vi "Update Data.vi"(3 "Data IN":T1={"PDFTable ref"=refnum, "columnWidth (points)"=[], "Borders"={"Row Borders [ ]"=[], "Last Row"={"Column Borders [ ]"=[], "Line"={"Thickness"=0.5, "Color"=0}}, "Row Back Ground color"={"color"=16777225, "at each"=0.0}}, "Image to Add with path[ ]"=[], "Image to Add with refnum[ ]"=[], "Update"=enum."Others"} caption="Data" {"Image to Add with path[ ]"."Scale" format="%#_g %"}) -> (0 "Data change?":bool, 1 "Data OUT":T1={"PDFTable ref"=refnum, "columnWidth (points)"=[], "Borders"={"Row Borders [ ]"=[], "Last Row"={"Column Borders [ ]"=[], "Line"={"Thickness"=0.5, "Color"=0}}, "Row Back Ground color"={"color"=16777225, "at each"=0.0}}, "Image to Add with path[ ]"=[], "Image to Add with refnum[ ]"=[], "Update"=enum."Others"} caption="Data" {"Image to Add with path[ ]"."Scale" format="%#_g %"})   [LabVIEW 2012]
uses:
  C:/Users/MaxCorp/Documents/GitHub/TopView/DLL/itextsharp.dll
  GitHub/TopView/DLL/itextsharp.dll
  Image Scale.ctl
  Cell Border.ctl
  <userlib>/Exaprom PDF/Controls/PDF Table Xcontrol/Data.ctl
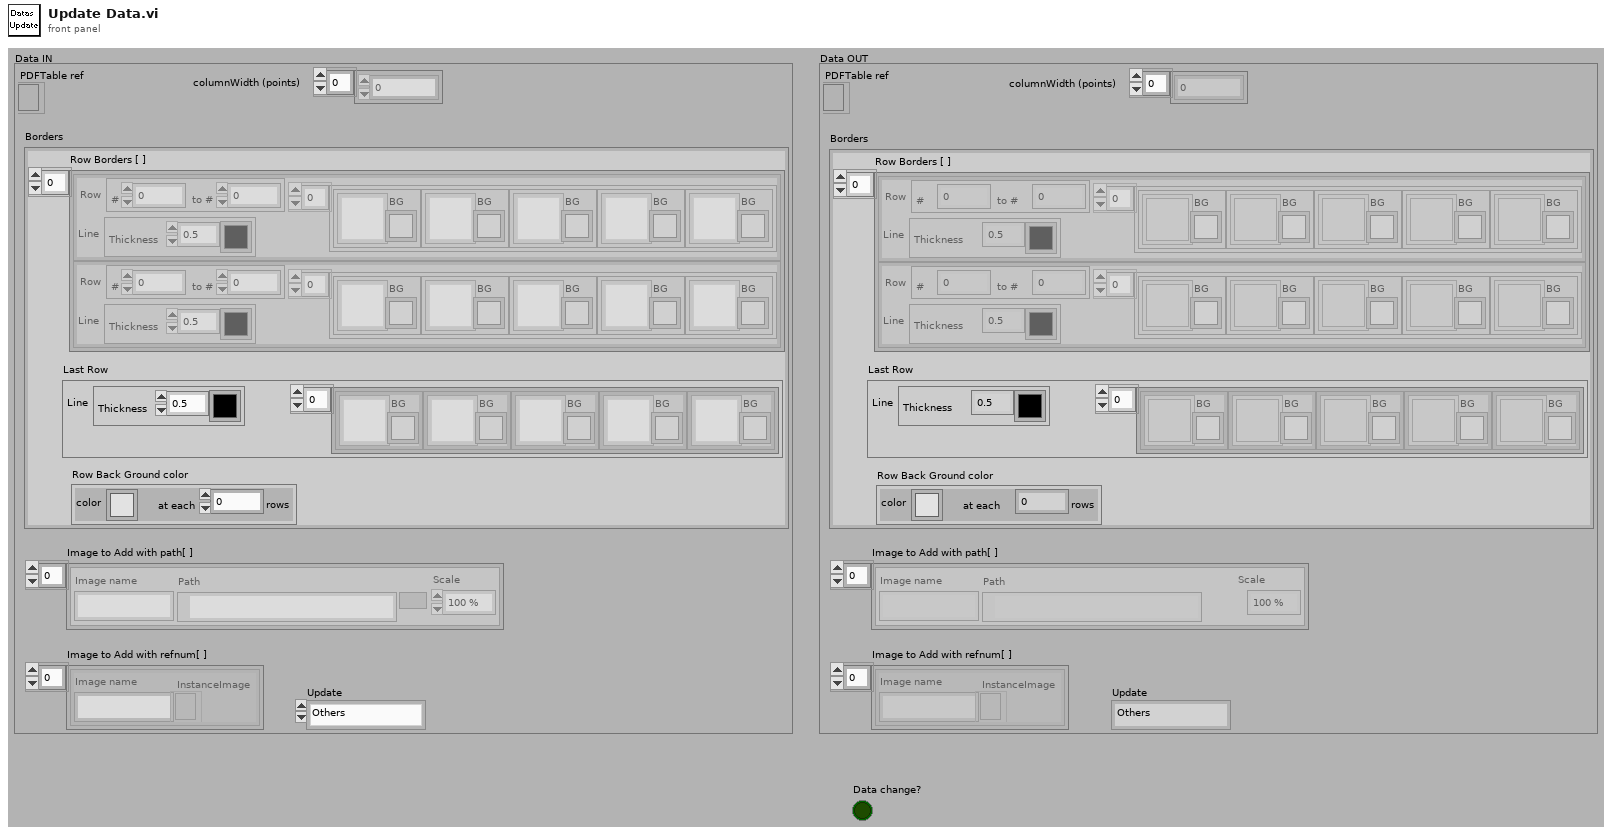
[diagram p1: front panel]
types:
  T1 = typedef "PDF Table XControl.xctl/Data.ctl" = cluster{"PDFTable ref":refnum<k24>, "columnWidth (points)":sgl[], "Borders":cluster{"Row Borders [ ]":cluster{"Column Borders [ ]":cluster{"Cell Border":T2, "BG":u32}[], "Line":cluster{"Thickness":sgl, "Color":u32}, "Row":cluster{"#":u16, "to #":i16}}[], "Last Row":cluster{"Column Borders [ ]":cluster{"Cell Border":T2, "BG":u32}[], "Line":cluster{"Thickness":sgl, "Color":u32}}, "Row Back Ground color":cluster{"color":u32, "at each":dbl}}, "Image to Add with path[ ]":cluster{"Image name":string, "Path":path, "Scale":T3}[], "Image to Add with refnum[ ]":cluster{"Image name":string, "InstanceImage":refnum<k24>}[], "Update":enum16{"Others", "Borders", "Images List"}}
  T2 = typedef "Cell Border.ctl" = u16
  T3 = typedef "Image Scale.ctl" = sgl
  T4 = cluster{"Image name":string, "InstanceImage":refnum<k24>}[]
  T5 = cluster{"Image name":string, "Path":path, "Scale":T3}[]
  T6 = cluster{"Image name":string, "GetInstance":refnum<k24>}
  T7 = cluster{"Image name":string, "GetInstance":refnum<k24>}[]
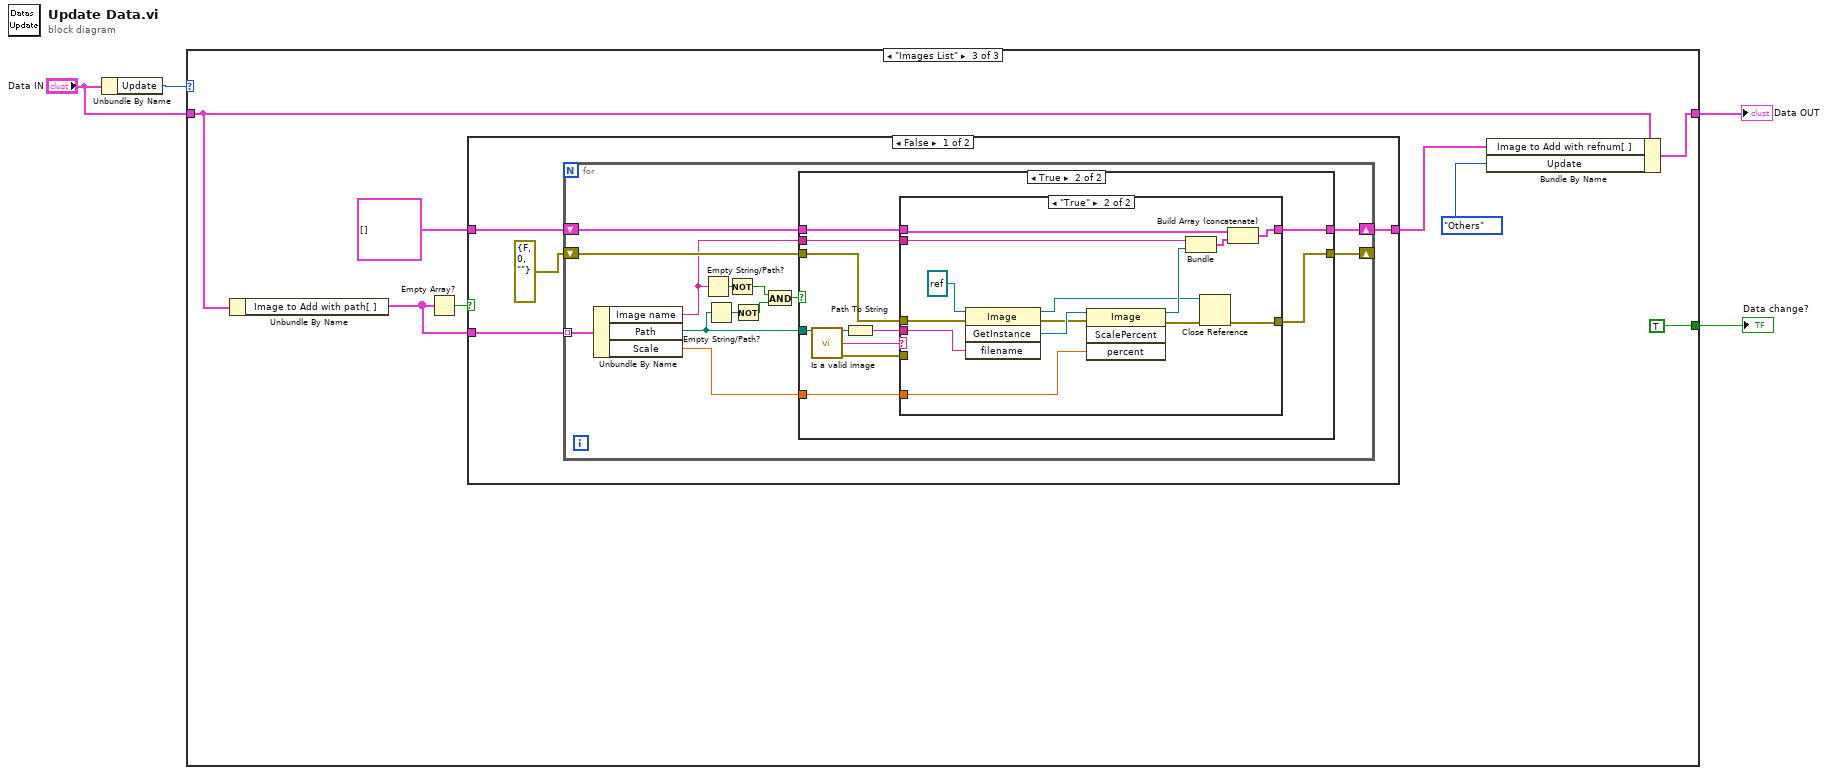
[diagram p0: block diagram]
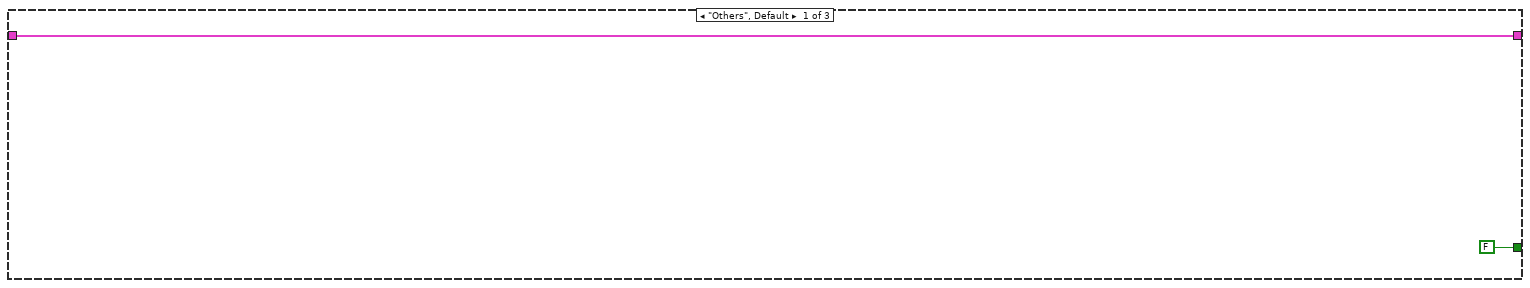
[diagram p2: hidden frame]
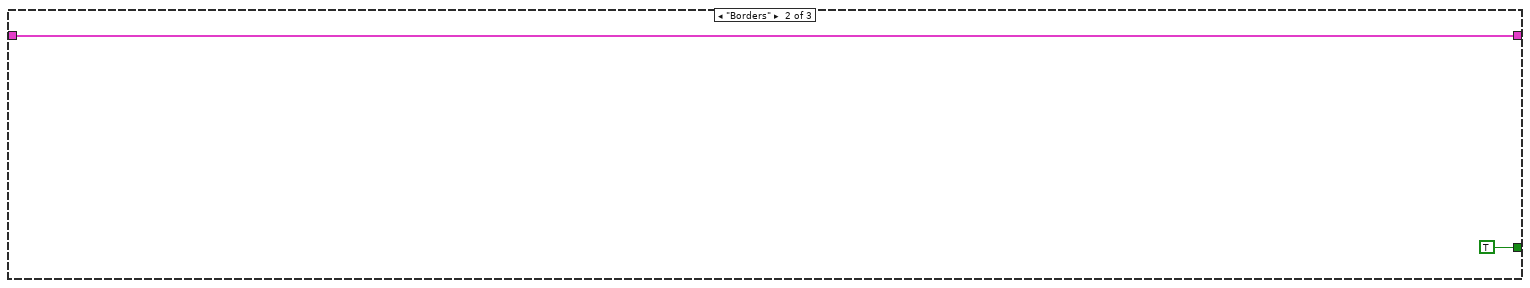
[diagram p3: hidden frame]
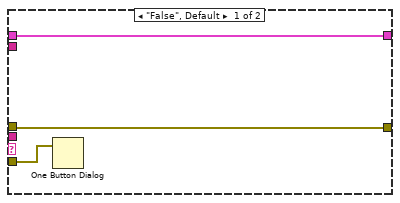
[diagram p5: hidden frame]
diagram:
  n1 = Unbundle By Name("Data IN") -> ("Update"=w4:enum16{"Others", "Borders", "Images List"})
  n2 = case shown="\"Images List\"" w4 {
    tunnel: "Data IN" -> [w6 w8 w12]
    tunnel: [w6 w8 w14] -> w2
    tunnel: [FALSE ("Data change?") TRUE ("Data change?") TRUE ("Data change?")] -> w1
    frame "Others", Default {
    }
    frame "Borders" {
    }
    frame "Images List" {
      n3 = Unbundle By Name(w12) -> ("Image to Add with path[ ]"=w11:T5)
      n4 = Empty Array?(array=w11) -> (empty?=w15:bool)
      n5 = case shown="False" w15 {
        tunnel: w11 -> [w20 _]
        tunnel: T4 [] ("Image to Add [ ]") -> [w19 w64]
        tunnel: [w18 w64] -> w13
        frame False {
          n6 = for {
            tunnel: w20 -> [w33] mode=indexing
            shift-right: [w26] -> w18
            shift-left: w19 -> [w27]
            shift-right: [w24] -> _
            shift-left: errorcluster {"status"=FALSE, "code"=0, "source"=""} ("error out") -> [w25]
            n7 = Unbundle By Name(w33) -> ("Image name"=w23:string, "Path"=w32:path, "Scale"=w28:T3)
            n8 = Empty String/Path?(string/path=w23) -> (empty?=w30:bool)
            n9 = Empty String/Path?(string/path=w32) -> (empty?=w31:bool)
            n10 = Not(x=w30) -> (.not. x?=w22:bool)
            n11 = Not(x=w31) -> (.not. x?=w21:bool)
            n12 = And(x=w22, y=w21) -> (x .and. y?=w29:bool)
            n13 = case shown="True" w29 {
              tunnel: w32 -> [_ w45]
              tunnel: w28 -> [_ w42]
              tunnel: w27 -> [w35 w39]
              tunnel: [w35 w38] -> w26
              tunnel: w25 -> [w34 w41]
              tunnel: [w34 w40] -> w24
              tunnel: w23 -> [_ w37]
              frame False {
              }
              frame True {
                n14 = call "Is a valid image.vi"("Image path"=w45) -> ("dup path"=w46:path, "Message"=w44:string, "error out"=w36:errorcluster)  [unwired: 1 in, 11 out]
                n15 = Path To String(path=w46) -> (string=w43:string)
                n16 = case shown="\"True\"" w44 {
                  tunnel: w43 -> [_ w61]
                  tunnel: w42 -> [_ w60]
                  tunnel: [w49 w52] -> w40
                  tunnel: w41 -> [w49 w59]
                  tunnel: w39 -> [w48 w58]
                  tunnel: [w48 w57] -> w38
                  tunnel: w37 -> [_ w55]
                  tunnel: w36 -> [w47 _]
                  frame "False", Default {
                    n17 = One Button Dialog(message=w47) -> ()  [unwired: 2 out]
                  }
                  frame "True" {
                    n18 = invoke class="Image" method="GetInstance"(reference=refnum<k24> refnum ("image"), error in=w59, "filename"=w61) -> (reference out=w51:refnum<k24>, error out=w62:errorcluster, "GetInstance"=w63:refnum<k24>)  [unwired: 1 in, 1 out]
                    n19 = invoke class="Image" method="ScalePercent"(reference=w63, error in=w62, "percent"=w60) -> (reference out=w56:refnum<k24>, error out=w53:errorcluster)  [unwired: 1 in, 2 out]
                    n20 = Bundle("Image name"=w55, "GetInstance"=w56) -> (w54:T6)  [unwired: 1 out]
                    n21 = Close Reference(reference=w51, error in (no error)=w53) -> (error out=w52:errorcluster)
                    n22 = Build Array (concatenate)(w58, w54) -> (w57:T7)
                  }
                }
              }
            }
          }
        }
        frame True {
        }
      }
      n23 = Bundle By Name(cluster=w12, "Image to Add with refnum[ ]"=w13, "Update"=enum16{"Others", "Borders", "Images List"}."Others") -> (w14:T1)
    }
  }
  "Data OUT" <- w2
  "Data change?" <- w1
